vi "Read.vi"(8 "error in (no error)":errorcluster, 11 "Simulated Oscilloscope in":refnum<class "Simulated Oscilloscope.lvclass">) -> (0 "error out":errorcluster, 1 "timed out?":bool, 2 "Data out":refnum<class "AbstractData.lvclass">, 3 "Simulated Oscilloscope out":refnum<class "Simulated Oscilloscope.lvclass">)   [LabVIEW 2014, in "Simulated Oscilloscope.lvclass"]
uses:
  Simulated Oscilloscope.lvclass
  Framework/Model/Data/AbstractData/AbstractData.lvclass
  Framework/Model/Data/Data1D/Data1D.lvclass
  Simulated Oscilloscope.lvclass/Simulated Oscilloscope.ctl
  Framework/Interfaces/Observable Actor/Observable Actor.lvclass
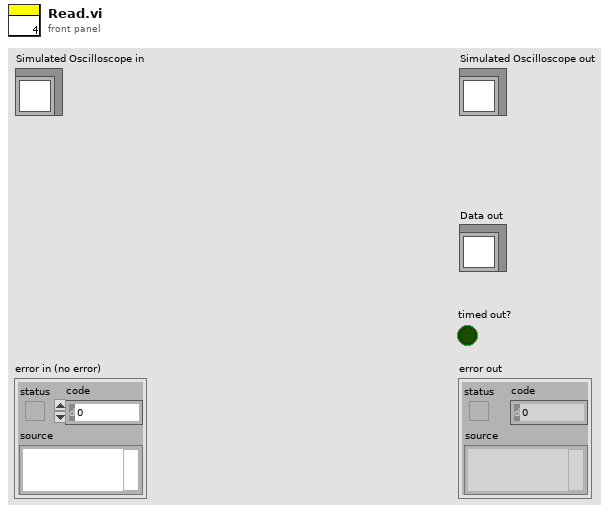
[diagram p1: front panel]
types:
  T1 = typedef "Simulated Oscilloscope.lvclass/Params.ctl" = cluster{"Amplitude":dbl, "Y Offset":dbl, "X Offset":dbl, "Period":dbl, "Ticks per frame":dbl, "Noise Amplitude":dbl, "dt":dbl}
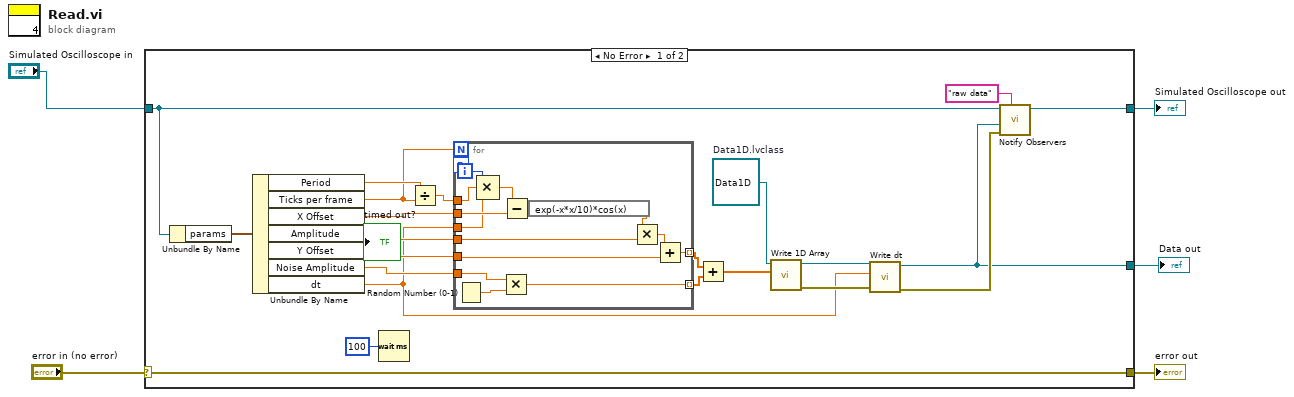
[diagram p0: block diagram]
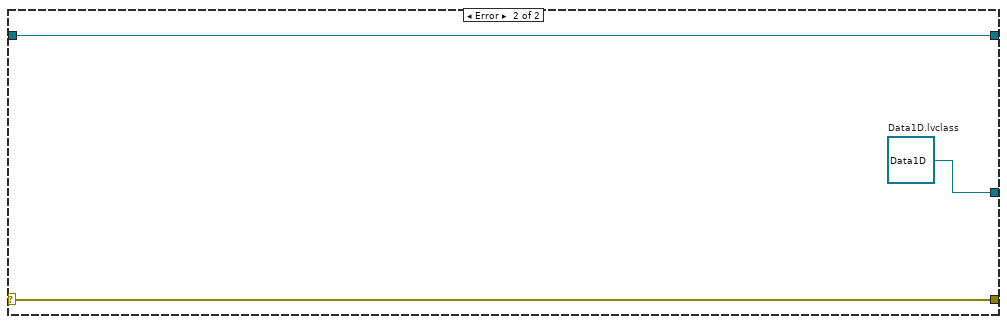
[diagram p2: hidden frame]
diagram:
  n1 = case shown="No Error" "error in (no error)" {
    selector: "error in (no error)" -> [w7 w44]
    tunnel: [w7 w44] -> w3
    tunnel: [w12 w43] -> w2
    tunnel: "Simulated Oscilloscope in" -> [w8 w43]
    tunnel: [w10 w42] -> w1
    frame No Error {
      w18 = refnum<class "Data1D.lvclass"> refnum  # Data1D.lvclass
      n2 = Unbundle By Name(w8) -> ("params"=w9:T1)
      n3 = Unbundle By Name(w9) -> ("Period"=w27:dbl, "Ticks per frame"=w21:dbl, "X Offset"=w25:dbl, "Amplitude"=w24:dbl, "Y Offset"=w22:dbl, "Noise Amplitude"=w23:dbl, "dt"=w14:dbl)
      n4 = Wait (ms)(milliseconds to wait=u32 100) -> ()  [unwired: 1 out]
      n5 = Divide(x=w27, y=w21) -> (x/y=w26:dbl)
      n6 = for {
        N: w21 -> [_]
        tunnel: w26 -> [w29]
        tunnel: w25 -> [w41]
        tunnel: w23 -> [w38]
        tunnel: w24 -> [w36]
        tunnel: [w32] -> w17 mode=indexing
        tunnel: [w35] -> w16 mode=indexing
        tunnel: w22 -> [w33]
        tunnel: w14 -> [w28]
        workers-P: _ -> [_]
        i -> [w31]
        n7 = Random Number (0-1)() -> (number: 0 to 1=w39:dbl)
        n8 = Compound Arithmetic op=MULTIPLY(w31, w29, w28) -> (w30:dbl)
        n9 = Multiply(x=w38, y=w39) -> (x*y=w35:dbl)
        n10 = Subtract(x=w30, y=w41) -> (x-y=w40:dbl)
        n11 = expression code="exp(-x*x/10)*cos(x)"(w40) -> (w37:dbl)
        n12 = Multiply(x=w37, y=w36) -> (x*y=w34:dbl)
        n13 = Add(x=w34, y=w33) -> (x+y=w32:dbl)
      }
      n14 = Add(x=w17, y=w16) -> (x+y=w15:dbl[])
      n15 = call "Write 1D Array.vi"("1D Array"=w15, "Data1D in"=w18) -> ("error out"=w19:errorcluster, "Data1D out"=w20:refnum<class "Data1D.lvclass">)  [unwired: 8 in]
      n16 = call "Write dt.vi"("error in (no error)"=w19, "dt"=w14, "Data1D in"=w20) -> ("error out"=w11:errorcluster, "Data1D out"=w10:refnum<class "Data1D.lvclass">)  [unwired: 7 in]
      n17 = call "Notify Observers.vi"("name"="raw data", "error in (no error)"=w11, "value"=w10, "Observable Actor in"=w8) -> ("Observable Actor out"=w12:refnum<class "Simulated Oscilloscope.lvclass">)  [unwired: 6 in, 1 out]
    }
    frame Error {
      w42 = refnum<class "Data1D.lvclass"> refnum  # Data1D.lvclass
    }
  }
  "error out" <- w3
  "Simulated Oscilloscope out" <- w2
  "Data out" <- w1
